vi "Stop Octave.vi"(6 "Stop Octave?":bool, 8 "error in (no error)":errorcluster, 11 "GOLPI ref. in":T1) -> (0 "error out":errorcluster, 3 "GOLPI ref. out":T1)   [LabVIEW 2020]
doc: "Stops Octave if input set to stop."
uses:
  external libraries/GOLPI 0.7.3.1 source distribution LV 20.0 32 bit/Pipe Handle.ctl
  external libraries/GOLPI 0.7.3.1 source distribution LV 20.0 32 bit/LV Process library.lvlib
  external libraries/GOLPI 0.7.3.1 source distribution LV 20.0 32 bit/GOLPI reference Type Def.ctl
  external libraries/GOLPI 0.7.3.1 source distribution LV 20.0 32 bit/GOLPI library.lvlib
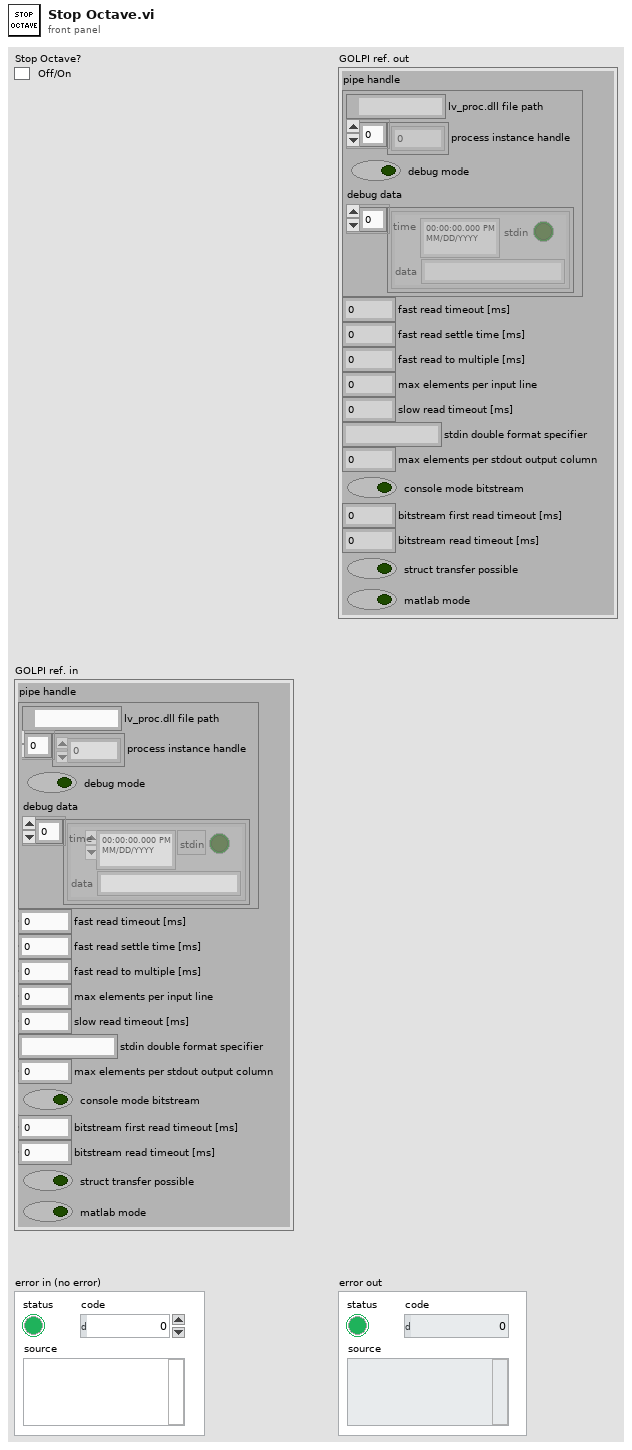
[diagram p1: front panel]
types:
  T1 = typedef "GOLPI library.lvlib/GOLPI reference Type Def.ctl" = cluster{"pipe handle":T2, "fast read timeout [ms]":u32, "fast read settle time [ms]":u32, "fast read to multiple [ms]":u32, "max elements per input line":u32, "slow read timeout [ms]":u32, "stdin double format specifier":string, "max elements per stdout output column":u32, "console mode bitstream":bool, "bitstream first read timeout [ms]":u32, "bitstream read timeout [ms]":u32, "struct transfer possible":bool, "matlab mode":bool}
  T2 = typedef "LV Process library.lvlib/Pipe Handle.ctl" = cluster{"lv_proc.dll file path":path, "process instance handle":u32[], "debug mode":bool, "debug data":cluster{"time":timestamp, "stdin":bool, "data":string}[]}
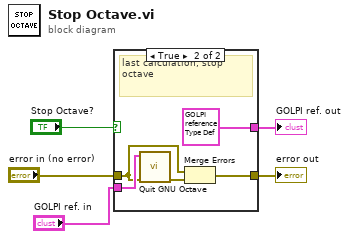
[diagram p0: block diagram]
diagram:
  n1 = case shown="True" "Stop Octave?" {
    tunnel: [w7 w8] -> w1
    tunnel: "error in (no error)" -> [w7 w9]
    tunnel: "GOLPI ref. in" -> [w6 w12]
    tunnel: [w6 T1 {"pipe handle"={"lv_proc.dll file path"=path "", "process instance handle"=[], "debug mode"=FALSE, "debug data"=[]}, "fast read timeout [ms]"=500, "fast read settle time [ms]"=10, "fast read to multiple [ms]"=1, "max elements per input line"=100, "slow read timeout [ms]"=5000, "stdin double format specifier"="%_16e", "max elements per stdout output column"=100, "console mode bitstream"=FALSE, "bitstream first read timeout [ms]"=1000, "bitstream read timeout [ms]"=50, "struct transfer possible"=FALSE, "matlab mode"=FALSE} ("GOLPI ref. out")] -> w5
    frame False {
    }
    frame True {
      # "last calculation, stop\noctave"
      n2 = call "Quit GNU Octave.vi"("error in"=w9, "GOLPI ref. in"=w12) -> ("error out"=w10:errorcluster)  [unwired: 8 in, 1 out]
      n3 = Merge Errors(w9, w10) -> (w8:errorcluster)
    }
  }
  "GOLPI ref. out" <- w5
  "error out" <- w1
